vi "Set regeneration.vi"(8 "error in (no error)":errorcluster, 10 "regeneration":bool, 11 "NI Analog Output in":refnum<class "NI Analog Output.lvclass">) -> (0 "error out":errorcluster, 3 "NI Analog Output out":refnum<class "NI Analog Output.lvclass">)   [LabVIEW 2020, in "NI DAQmx.lvlib" / "NI Analog Output.lvclass"]
uses:
  NI Analog Output.lvclass
  NI Analog Output.lvclass/NI Analog Output.ctl
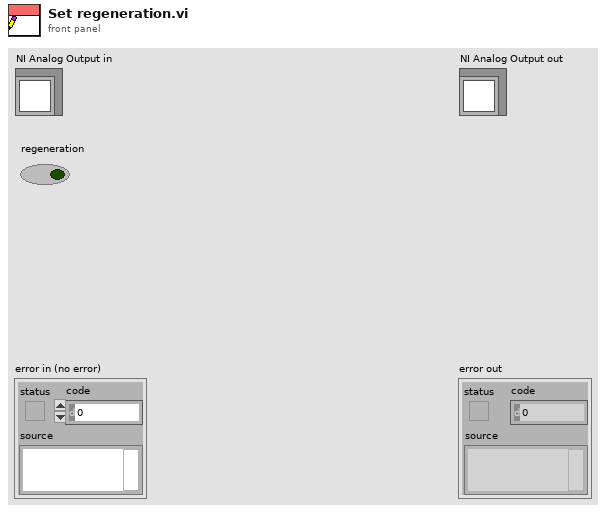
[diagram p1: front panel]
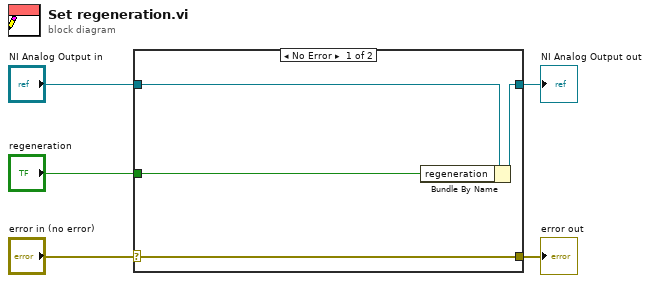
[diagram p0: block diagram]
diagram:
  n1 = case shown="No Error" "error in (no error)" {
    selector: "error in (no error)" -> [w9 w10]
    tunnel: [w9 w10] -> w4
    tunnel: [w7 w11] -> w2
    tunnel: "NI Analog Output in" -> [w8 w11]
    tunnel: "regeneration" -> [w6 _]
    frame No Error {
      n2 = Bundle By Name(cluster=w8, "regeneration"=w6) -> (w7:refnum<class "NI Analog Output.lvclass">)
    }
    frame Error {
    }
  }
  "error out" <- w4
  "NI Analog Output out" <- w2
